vi "Voltage Multiplu Measurements.vi"() -> ()   [LabVIEW 2013]
uses:
  <vilib>/Analysis/baseanly.llb/Mean (DBL).vi
  <vilib>/Utility/file.llb/Write To Spreadsheet File (DBL).vi
  <vilib>/Analysis/NI_AALBase.lvlib
panel:
  in  "Write report":bool
  in  "File Path":path
  out "VOltage Array":dbl[](array[numeric])
  out "Waveform Graph":cluster{i32, dbl, dbl[]}(graph)
  out "Waveform Chart":dbl(graph)
  out "AVG, V":dbl
  out "Min Value, V":dbl
  out "Max Value, V":dbl
  in  "Number of samples":i32
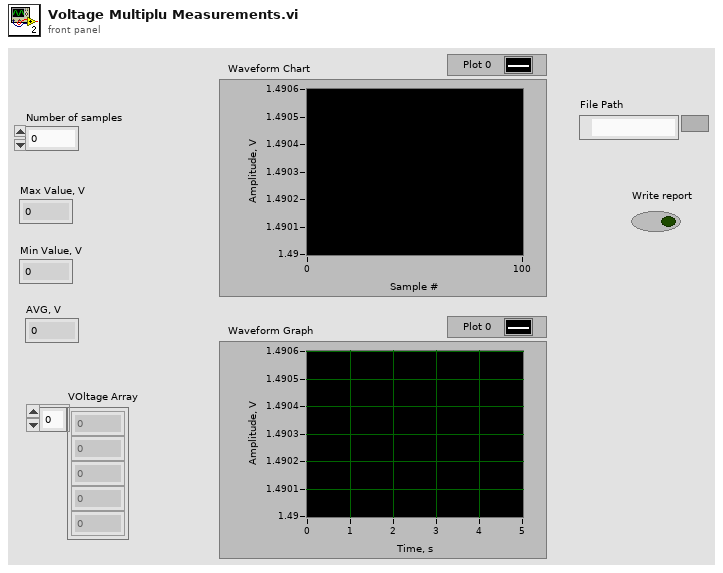
[diagram p1: front panel]
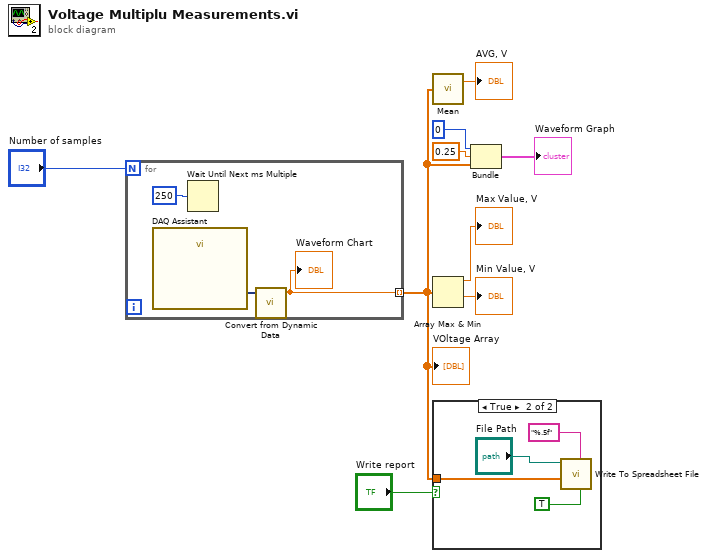
[diagram p0: block diagram]
diagram:
  n1 = for {
    N: "Number of samples" -> [_]
    tunnel: [w10] -> w1 mode=indexing
    n2 = call "DAQ Assistant"() -> ("data"=w11:dynamicdata)  [unwired: 17 in, 2 out]
    n3 = Wait Until Next ms Multiple(millisecond multiple=u32 250) -> ()  [unwired: 1 out]
    n4 = call "Convert from Dynamic Data"("Dynamic Data Type"=w11) -> ("Scalar"=w10:dbl)  [unwired: 3 in]
    "Waveform Chart" <- w10
  }
  "VOltage Array" <- w1
  n5 = call-poly <vilib>:"Mean.vi"("X"=w1) -> ("mean"=→"AVG, V":dbl)  [unwired: 1 out]
  n6 = Array Max & Min(array=w1) -> (max value=→"Max Value, V":dbl, min value=→"Min Value, V":dbl)  [unwired: 2 out]
  n7 = case shown="True" "Write report" {
    tunnel: w1 -> [_ w15]
    frame False {
    }
    frame True {
      n8 = call-poly <vilib>:"Write To Spreadsheet File.vi"("transpose? (no:F)"=TRUE, "format (%.3f)"="%.5f", "1D data"=w15, "file path (dialog if empty)"="File Path") -> ()  [unwired: 4 in, 1 out]
    }
  }
  n9 = Bundle(0, 0.25, w1) -> (→"Waveform Graph":cluster{i32, dbl, dbl[]})  [unwired: 1 in]
